vi "Log debbug message.vi"(8 "error in (no error)":errorcluster, 10 "String":string, 11 "Channel in":refnum<class "Channel.lvclass">) -> (0 "error out":errorcluster, 3 "Channel out":refnum<class "Channel.lvclass">)   [LabVIEW 2018, in "Channel.lvclass"]
uses:
  Channel.lvclass
  Channel.lvclass/Channel.ctl
  Log File/Log File.lvclass
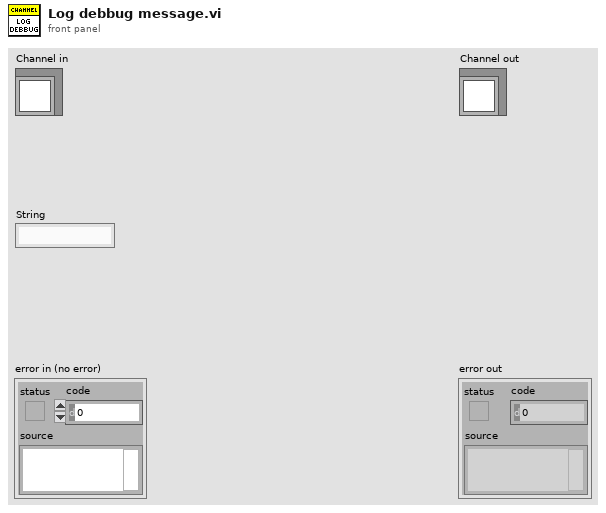
[diagram p1: front panel]
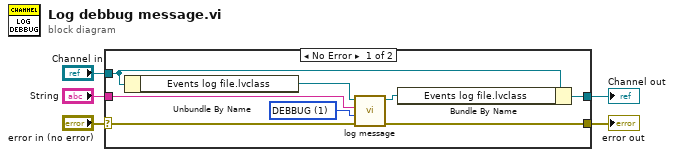
[diagram p0: block diagram]
diagram:
  n1 = case shown="No Error" "error in (no error)" {
    selector: "error in (no error)" -> [w9 w15]
    tunnel: [w8 w15] -> w4
    tunnel: [w10 w14] -> w2
    tunnel: "Channel in" -> [w11 w14]
    tunnel: "String" -> [w7 _]
    frame No Error {
      w6 = u16 1 items=[" STATUS ", " DEBBUG ", "  INFO  ", "WARNING ", " ERROR  ", "CRITICAL"] ("log level")
      n2 = Unbundle By Name(w11) -> ("Events log file.lvclass"=w13:refnum<class "Log File.lvclass">)
      n3 = call-dynamic "log message.vi"("error in (no error)"=w9, "log level"=w6, "Message to log"=w7, "Log File in"=w13) -> ("error out"=w8:errorcluster, "Log File out"=w12:refnum<class "Log File.lvclass">)  [unwired: 6 in]
      n4 = Bundle By Name(cluster=w11, "Events log file.lvclass"=w12) -> (w10:refnum<class "Channel.lvclass">)
    }
    frame Error {
    }
  }
  "error out" <- w4
  "Channel out" <- w2
